vi "TODO Write time series variant.vi"(0 "Client.lvclass in":refnum<class "Client.lvclass">, 5 "Database name":string, 7 "Series name":string, 9 "Precision":T1=enum."Milliseconds", 11 "error in (no error)":errorcluster, 12 "Variant data":variant) -> (4 "Client.lvclass out":refnum<class "Client.lvclass">, 15 "error out":errorcluster)   [LabVIEW 2018, in "InfluxDB Client.lvlib" / "Client.lvclass"]
doc: "Writes time series data (Variant format) to a specific database."
uses:
  Client.lvclass
  Controls/Precision.ctl
  Client.lvclass/Client.ctl
  <vilib>/httpClient/POSTBuffer.vi
  <vilib>/httpClient/LabVIEWHTTPClient.lvlib
  InfluxDB Client.lvlib
panel:
  out "Status":string
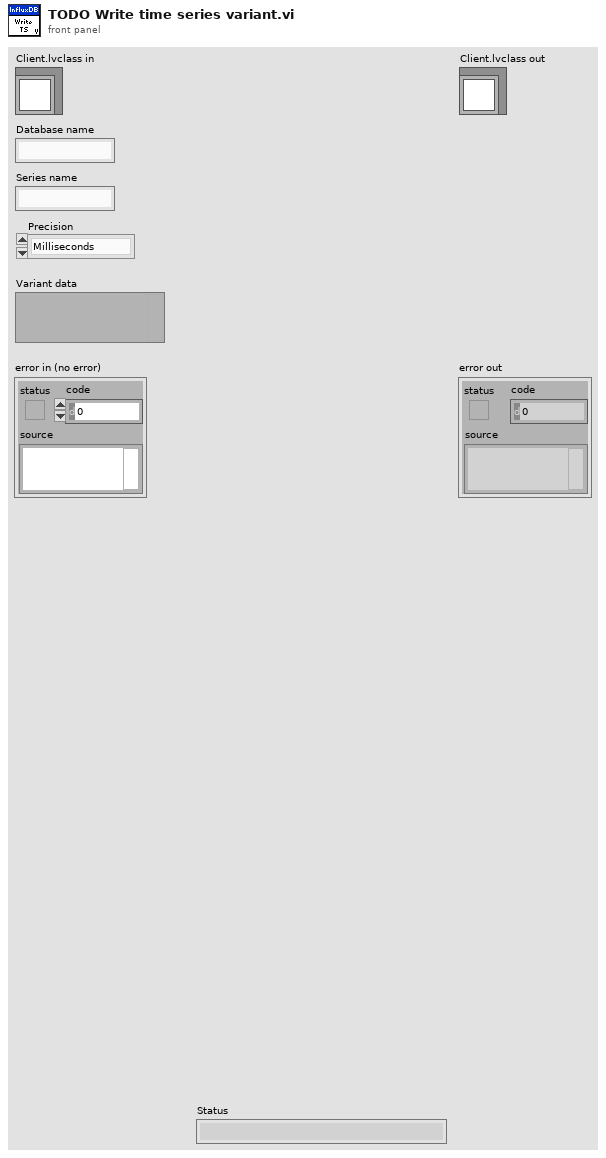
[diagram p1: front panel]
types:
  T1 = typedef "InfluxDB Client.lvlib/Precision.ctl" = enum16{"Seconds", "Milliseconds", "Nanoseconds"}
  T2 = typedef "LabVIEWHTTPClient.lvlib/ClientHandle.ctl" = refnum<k1>
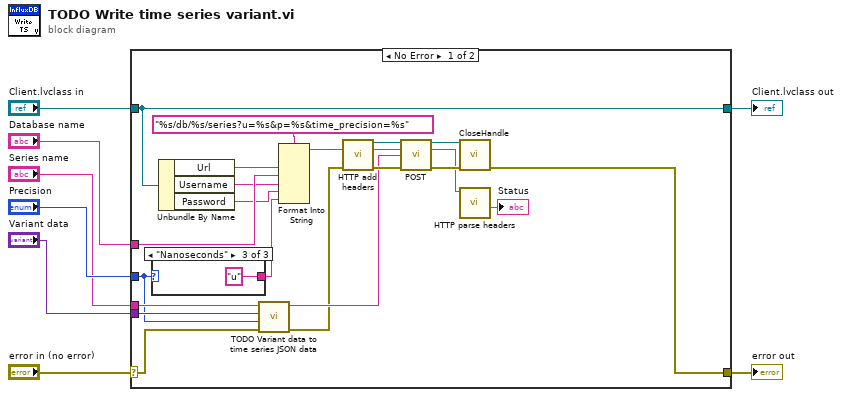
[diagram p0: block diagram]
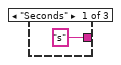
[diagram p2: hidden frame]
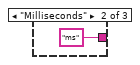
[diagram p3: hidden frame]
diagram:
  n1 = case shown="No Error" "error in (no error)" {
    selector: "error in (no error)" -> [w10 w34]
    tunnel: [w23 w34] -> w7
    tunnel: [w29 w33] -> w5
    tunnel: "Client.lvclass in" -> [w29 w33]
    tunnel: "Database name" -> [w20 _]
    tunnel: "Precision" -> [w11 _]
    tunnel: "Variant data" -> [w12 _]
    tunnel: "Series name" -> [w14 _]
    frame No Error {
      n2 = case shown="\"Nanoseconds\"" w11 {
        tunnel: ["s" ("Database name") "ms" ("Database name") "u" ("Database name")] -> w15
        frame "Seconds" {
        }
        frame "Milliseconds" {
        }
        frame "Nanoseconds" {
        }
      }
      n3 = Unbundle By Name(w29) -> ("Url"=w27:string, "Username"=w19:string, "Password"=w18:string)
      n4 = call "TODO Variant data to time series JSON data.vi"("error in (no error)"=w10, "Precision"=w11, "Data"=w12, "Series name"=w14) -> ("error out"=w9:errorcluster, "JSON data"=w13:string)  [unwired: 6 in]
      n5 = Format Into String(format string="%s/db/%s/series?u=%s&p=%s&time_precision=%s" ("url"), w27, w20, w19, w18, w15) -> (resulting string=w24:string)  [unwired: 2 in, 1 out]
      n6 = call "HTTP add headers.vi"("error in (no error)"=w9) -> ("client handle out"=w16:T2, "error out"=w17:errorcluster)  [unwired: 13 in]
      n7 = call-poly <vilib>:"POST.vi"("client handle"=w16, "url"=w24, "buffer"=w13, "error in (no error)"=w17) -> ("client handle out"=w26:T2, "headers"=w22:string, "error out"=w25:errorcluster)  [unwired: 8 in, 1 out]
      n8 = call <vilib>:"CloseHandle.vi"("client handle"=w26, "error in (no error)"=w25) -> ("error out"=w23:errorcluster)  [unwired: 13 in]
      n9 = call "HTTP parse headers.vi"("HTTP headers"=w22) -> ("Status"=→"Status":string)  [unwired: 7 in, 3 out]
    }
    frame Error {
    }
  }
  "error out" <- w7
  "Client.lvclass out" <- w5
